vi "BackwardsPropagation.vi"(6 "Array 4":dbl[](array[numeric]), 9 "Array 3":dbl[](array[numeric]), 10 "Array in":cluster{dbl[]}[](array[cluster]), 11 "Array 5":cluster{"A - B":T1}[](array[cluster])) -> (2 "Array":cluster{"Outer Product":T1}[](array[cluster]), 3 "Array 2":cluster{"A - B":T1}[](array[cluster]))   [LabVIEW 2016]
uses:
  <vilib>/Analysis/Matrix/Datatypes/RealMatrix.ctl
  <vilib>/Analysis/baseanly.llb/Vector x A.vi
  <vilib>/Analysis/baseanly.llb/Real Outer Product.vi
  <vilib>/Analysis/Matrix/Numeric/Multiply/Multiply - RM,R.vi
  <vilib>/Analysis/Matrix/Numeric/Subtract/Subtract - RM,RM.vi
  <vilib>/Analysis/NI_AALBase.lvlib
  <vilib>/Analysis/Matrix/NI_Matrix.lvlib
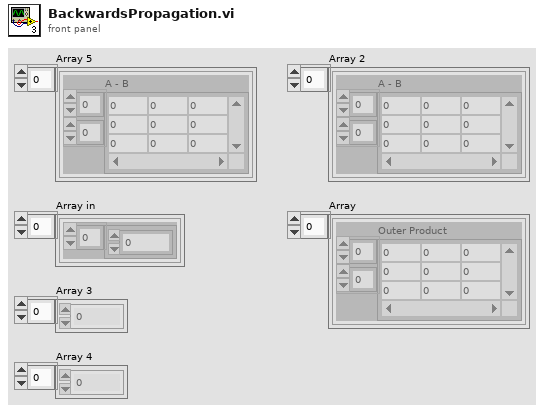
[diagram p1: front panel]
types:
  T1 = typedef "NI_Matrix.lvlib/RealMatrix.ctl" = dbl[][]
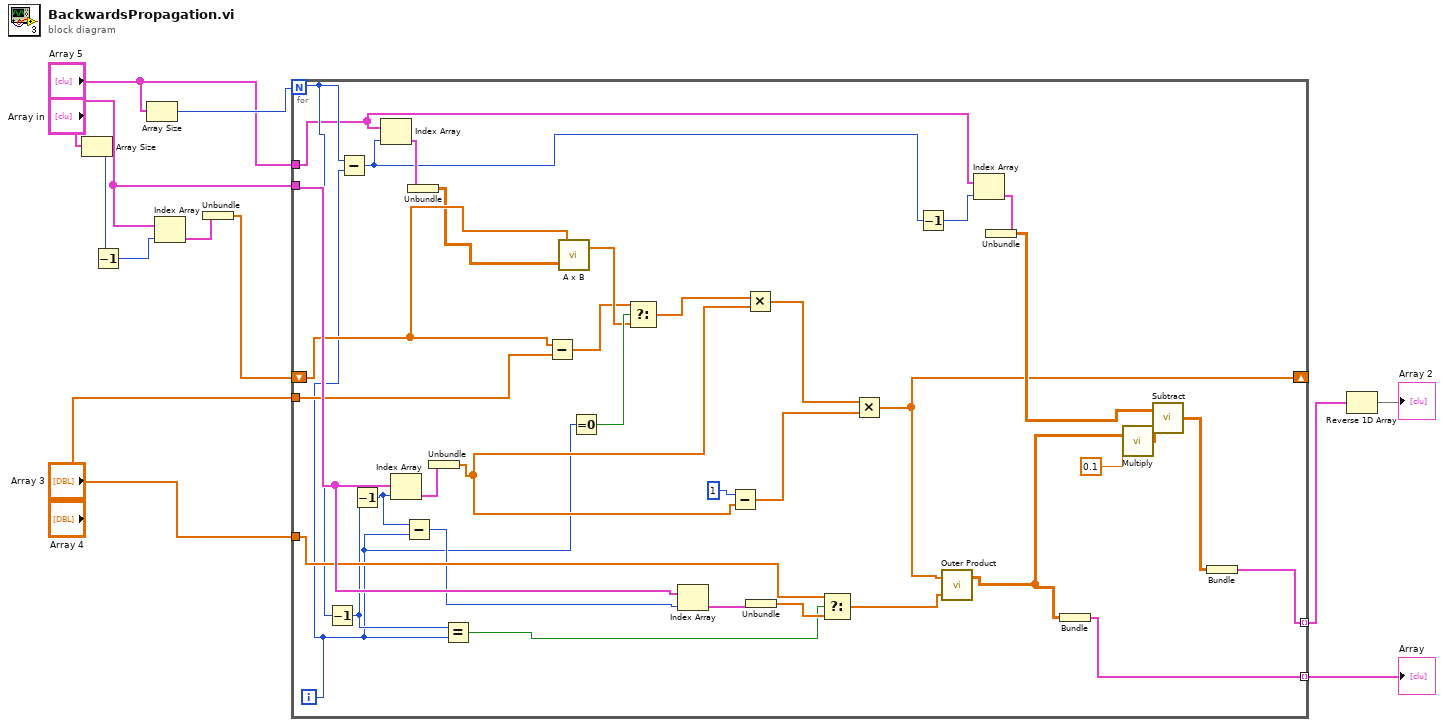
[diagram p0: block diagram]
diagram:
  n1 = Array Size(array="Array in") -> (size(s)=w2:i32)
  n2 = Decrement(x=w2) -> (x-1=w3:i32)
  n3 = Array Size(array="Array 5") -> (size(s)=w6:i32)
  n4 = Index Array(array="Array in", index=w3) -> (element=w1:cluster{dbl[]})
  n5 = Unbundle(w1) -> (w7:dbl[])
  n6 = for {
    N: w6 -> [w28]
    tunnel: "Array 5" -> [w24]
    tunnel: "Array in" -> [w48]
    tunnel: "Array 3" -> [w47]
    shift-right: [w19] -> _
    shift-left: w7 -> [w36]
    tunnel: "Array 4" -> [w35]
    tunnel: [w14] -> w11 mode=indexing
    tunnel: [w13] -> w12 mode=indexing
    i -> [w27]
    n7 = Decrement(x=w28) -> (x-1=w29:i32)
    n8 = Subtract(x=w28, y=w27) -> (x-y=w26:i32)
    n9 = Decrement(x=w29) -> (x-1=w38:i32)
    n10 = Index Array(array=w24, index=w26) -> (element=w46:cluster{"A - B":T1})
    n11 = Index Array(array=w48, index=w38) -> (element=w43:cluster{dbl[]})
    n12 = Subtract(x=w38, y=w27) -> (x-y=w37:i32)
    n13 = Unbundle(w46) -> ("A - B"=w30:T1)
    n14 = Unbundle(w43) -> (w42:dbl[])
    n15 = Equal?(x=w29, y=w27) -> (x = y?=w39:bool)
    n16 = Subtract(x=w36, y=w35) -> (x-y=w32:dbl[])
    n17 = call-poly <vilib>:"A x B.vi"("Matrix A"=w30, "Vector V'"=w36) -> ("V' x A"=w33:dbl[])  [unwired: 1 out]
    n18 = Equal To 0?(x=w27) -> (x = 0?=w34:bool)
    n19 = Select(t=w32, s=w34, f=w33) -> (s? t:f=w31:dbl[])
    n20 = Index Array(array=w48, index=w37) -> (element=w45:cluster{dbl[]})
    n21 = Subtract(x=1, y=w42) -> (x-y=w41:dbl[])
    n22 = Multiply(x=w31, y=w42) -> (x*y=w44:dbl[])
    n23 = Unbundle(w45) -> (w40:dbl[])
    n24 = Select(t=w47, s=w39, f=w40) -> (s? t:f=w20:dbl[])
    n25 = Multiply(x=w44, y=w41) -> (x*y=w19:dbl[])
    n26 = Decrement(x=w26) -> (x-1=w25:i32)
    n27 = call-poly <vilib>:"Outer Product.vi"("Y Vector"=w20, "X Vector"=w19) -> ("Outer Product"=w18:T1)  [unwired: 1 out]
    n28 = Index Array(array=w24, index=w25) -> (element=w23:cluster{"A - B":T1})
    n29 = Unbundle(w23) -> ("A - B"=w21:T1)
    n30 = Bundle("Outer Product"=w18) -> (w13:cluster{"Outer Product":T1})  [unwired: 1 in]
    n31 = call-poly <vilib>:"Multiply.vi"("Real Scalar c"=0.1, "Real Matrix A"=w18) -> ("A * c"=w16:T1)
    n32 = call-poly <vilib>:"Subtract.vi"("Real Matrix B"=w16, "Real Matrix A"=w21) -> ("A - B"=w22:T1)
    n33 = Bundle("A - B"=w22) -> (w14:cluster{"A - B":T1})  [unwired: 1 in]
  }
  "Array" <- w12
  n34 = Reverse 1D Array(array=w11) -> (reversed array=→"Array 2":cluster{"A - B":T1}[])
